vi "CheckIfStorageSizeExceeded.vi"(11 "BotResources":T1) -> (3 "FolderSizeExceeded":bool)   [LabVIEW 2015, in "TronviewGame.lvlib" / "Game.lvclass"]
uses:
  Game.lvclass
  TronVIEWBotAPI/BotData.ctl
  TronVIEWBotAPI/TronVIEWBotAPI.lvlib
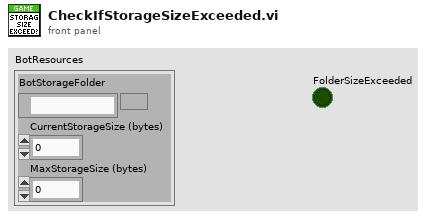
[diagram p1: front panel]
types:
  T1 = typedef "TronVIEWBotAPI.lvlib/BotData.ctl" = cluster{"BotStorageFolder":path, "CurrentStorageSize (bytes)":i64, "MaxStorageSize (bytes)":i64}
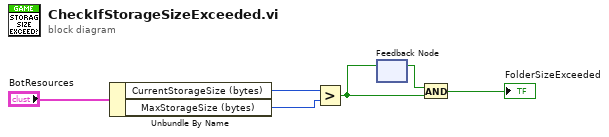
[diagram p0: block diagram]
diagram:
  n1 = Unbundle By Name("BotResources") -> ("CurrentStorageSize (bytes)"=w5:i64, "MaxStorageSize (bytes)"=w4:i64)
  n2 = Greater?(x=w5, y=w4) -> (0:w2:bool)
  n3 = feedback-in #1(w2) -> ()
  n4 = feedback #1() -> (w3:bool)  [unwired: 1 in]
  n5 = And(x=w3, y=w2) -> (x .and. y?=→"FolderSizeExceeded":bool)
